vi "FPGA SPI_Configure.vi"(7 "Hardware Pins":cluster{"RESET":bool, "LDAC":bool, "CLR":bool}, 8 "error in":errorcluster, 9 "Configuration Cluster":T1={"CS"=1, "Clock Rate (Hz)"=50000.0, "Clock Mode"=0, "CS Active State"=FALSE} {"CS" items=["0"=1, "1"=2, "2"=4, "3"=8, "4"=16, "5"=32, "6"=64, "7"=128]; "Clock Mode" items=["0", "1", "2", "3"]}, 10 "Port":i8, 11 "FPGA Interface":refnum<k20>) -> (0 "error out":errorcluster, 2 "Actual Rate (Hz)":dbl, 3 "FPGA VI Reference Out":refnum<k20>)   [LabVIEW 2014]
uses:
  <vilib>/rvi/interface/nirviReadWriteControl/nirviReadWriteControl.xnode
  DAC/Controls/FPGA SPI_FPGA SPI State.ctl
  FPGA Bitfiles/SPIExample_FPGATarget3_FPGASPIFPGATopLe_SKx8rjJlgp0.lvbitx
  FPGA/FPGA SPI_FPGA Top Level.vi
  Controls/SPI Configuration Cluster.ctl
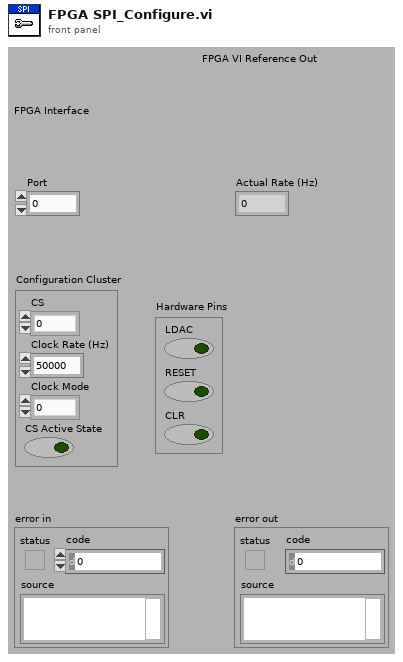
[diagram p1: front panel]
types:
  T1 = typedef "SPI Configuration Cluster.ctl" = cluster{"CS":u8, "Clock Rate (Hz)":dbl, "Clock Mode":u8, "CS Active State":bool}
  T2 = typedef "FPGA SPI_FPGA SPI State.ctl" = enum8{"Idle", "Read/Write SPI", "Configure"}
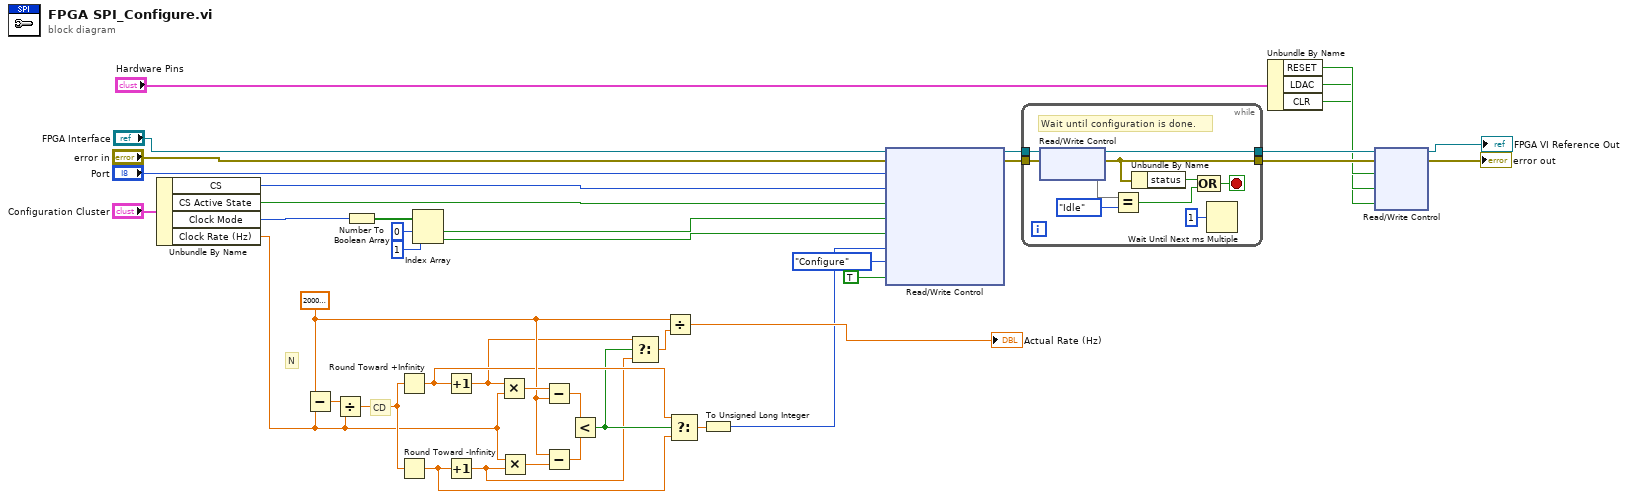
[diagram p0: block diagram]
diagram:
  w33 = 20000000.0 ("10M")
  # "CD"
  # "N"
  n1 = Unbundle By Name("Configuration Cluster") -> ("CS"=w38:u8, "CS Active State"=w15:bool, "Clock Mode"=w16:u8, "Clock Rate (Hz)"=w22:dbl)
  n2 = Subtract(x=w33, y=w22) -> (x-y=w32:dbl)
  n3 = Divide(x=w32, y=w22) -> (x/y=w31:dbl)
  n4 = Number To Boolean Array(number=w16) -> (Boolean array=w21:bool[])
  n5 = Round Toward +Infinity(x=w31) -> (ceil(x): smallest int >= x=w30:dbl)
  n6 = Round Toward -Infinity(1:w31) -> (0:w29:dbl)
  n7 = Index Array(array=w21, index #1=0 ("index"), index #2=1 ("index")) -> (element #1=w18:bool, element #2=w17:bool)
  n8 = Increment(x=w30) -> (x+1=w25:dbl)
  n9 = Increment(x=w29) -> (x+1=w26:dbl)
  n10 = Multiply(x=w25, y=w22) -> (x*y=w37:dbl)
  n11 = Multiply(x=w22, y=w26) -> (x*y=w36:dbl)
  n12 = Subtract(x=w37, y=w33) -> (x-y=w34:dbl)
  n13 = Subtract(x=w33, y=w36) -> (x-y=w35:dbl)
  n14 = Less?(x=w34, y=w35) -> (x < y?=w27:bool)
  n15 = Select(t=w25, s=w27, f=w26) -> (s? t:f=w28:dbl)
  n16 = Divide(x=w33, y=w28) -> (x/y=→"Actual Rate (Hz)":dbl)
  n17 = Select(t=w30, s=w27, f=w29) -> (s? t:f=w23:dbl)
  n18 = To Unsigned Long Integer(number=w23) -> (unsigned 32bit integer=w14:u32)
  n19 = xnode "Read/Write Control"("FPGA VI Reference In"="FPGA Interface", "error in"="error in", "SPI_Port"="Port", "SPI_CS"=w38, "SPI_CS Active State"=w15, "SPI_CPHA"=w18, "SPI_CPOL"=w17, "SPI_Clock Divider"=w14, "SPI_Cmd"=FPGA_SPI_FPGA_SPI_State."Configure" ("Cmd"), "SPI_Start"=TRUE ("Start")) -> ("FPGA VI Reference Out"=w11:refnum<k20>, "error out"=w10:errorcluster)
  n20 = while {
    tunnel: w11 -> [w51]
    tunnel: [w50] -> w9
    tunnel: w10 -> [w49]
    tunnel: [w46] -> w7
    stop <- w43 stop-if-true
    # "Wait until configuration is done."
    n21 = xnode "Read/Write Control"("FPGA VI Reference In"=w51, "error in"=w49) -> ("FPGA VI Reference Out"=w50:refnum<k20>, "error out"=w46:errorcluster, "SPI_Cmd"=w48)
    n22 = Equal?(x=w48, y=FPGA_SPI_FPGA_SPI_State."Idle") -> (x = y?=w44:bool)
    n23 = Unbundle By Name(w46) -> ("status"=w45:bool)
    n24 = Compound Arithmetic op=OR(w45, w44) -> (w43:bool)
    n25 = Wait Until Next ms Multiple(millisecond multiple=u32 1) -> ()  [unwired: 1 out]
  }
  n26 = Unbundle By Name("Hardware Pins") -> ("RESET"=w4:bool, "LDAC"=w3:bool, "CLR"=w2:bool)
  n27 = xnode "Read/Write Control"("FPGA VI Reference In"=w9, "error in"=w7, "RESET"=w4, "LDAC"=w3, "CLR"=w2) -> ("FPGA VI Reference Out"=→"FPGA VI Reference Out":refnum<k20>, "error out"=→"error out":errorcluster)
